vi "Acquire.vi"(8 "error in (no error)":errorcluster, 9 "Data Queue":refnum<queue>, 10 "Data Notifier":refnum<notifier>, 11 "Hardware Resources in":T1) -> (0 "error out":errorcluster, 3 "Hardware Resources out":T1)   [LabVIEW 2016, in "Acquisition.lvlib"]
doc: "Perform the acquisition. Replace the contents of this diagram with calls to acquisition hardware."
uses:
  Acquisition.lvlib
  Hardware Configuration.ctl
  <vilib>/DAQmx/read.llb/DAQmx Read (Analog 1D Wfm NChan NSamp).vi
  <vilib>/DAQmx/miscellaneous.llb/DAQmx Fill In Error Info.vi
  <resource>/objmgr/daqmx.rc
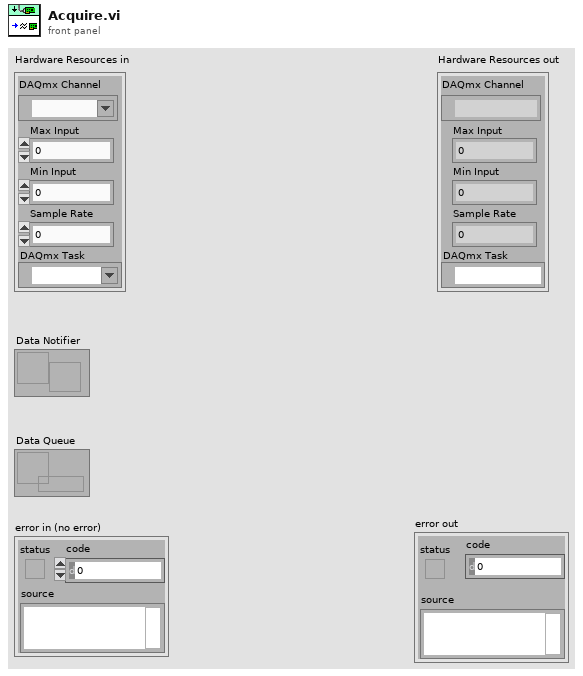
[diagram p1: front panel]
types:
  T1 = typedef "Acquisition.lvlib/Hardware Configuration.ctl" = cluster{"DAQmx Channel":tag, "Max Input":dbl, "Min Input":dbl, "Sample Rate":dbl, "DAQmx Task":refnum<k21>}
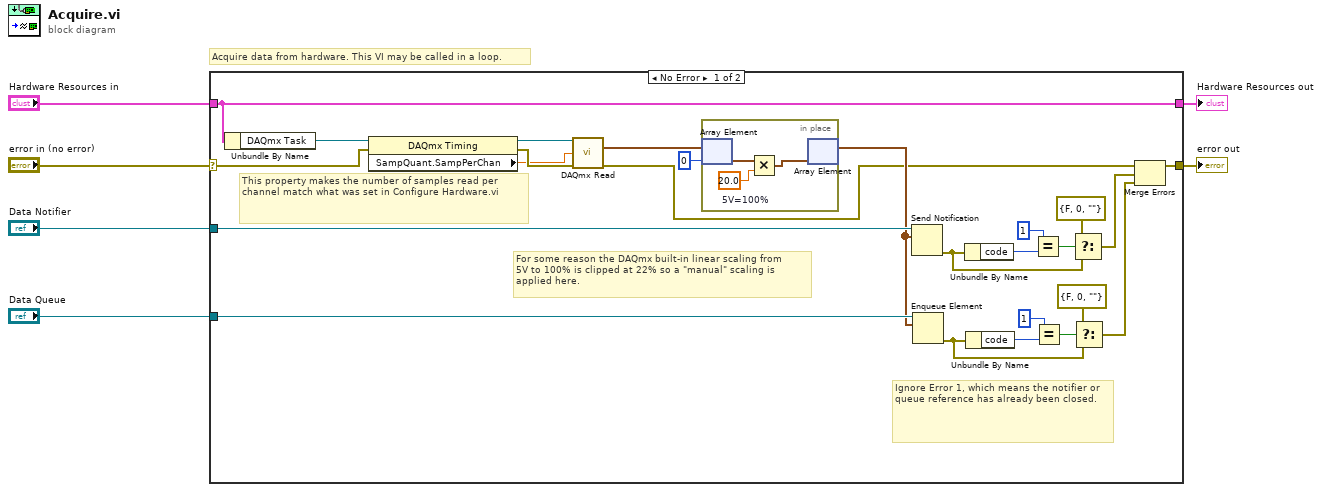
[diagram p0: block diagram]
diagram:
  # "Acquire data from hardware. This VI may be called in a loop."
  n1 = case shown="No Error" "error in (no error)" {
    selector: "error in (no error)" -> [w13 w35]
    tunnel: [w31 w35] -> w5
    tunnel: "Hardware Resources in" -> [w16 w36]
    tunnel: [w16 w36] -> w3
    tunnel: "Data Notifier" -> [w30 _]
    tunnel: "Data Queue" -> [w17 _]
    frame No Error {
      # "For some reason the DAQmx built-in linear scaling from\n5V to 100% is clipped at 22% so a \"manual\" scaling is\napplied here."
      # "This property makes the number of samples read per channel match what was set in Configure Hardware.vi"
      # "Ignore Error 1, which means the notifier or queue reference has already been closed."
      n2 = Unbundle By Name(w16) -> ("DAQmx Task"=w15:refnum<k21>)
      n3 = property class="DAQmx Timing"(reference=w15, error in=w13) -> (reference out=w14:refnum<k21>, error out=w12:errorcluster, "SampQuant.SampPerChan"=w11:dbl)
      n4 = call-poly <vilib>:"DAQmx Read.vi"("task/channels in"=w14, "number of samples per channel"=w11, "error in"=w12) -> ("data"=w9:waveform(dbl)[], "error out"=w7:errorcluster)  [unwired: 10 in, 1 out]
      n5 = in-place {
        w33 = 20.0  # 5V=100%
        n6 = in-place-array #1(w9, 0) -> (w34:waveform(dbl))
        n7 = Multiply(x=w34, y=w33) -> (x*y=w32:waveform(dbl))
        n8 = in-place-array #1(w32) -> (w8:waveform(dbl)[])  [unwired: 1 out]
      }
      n9 = Send Notification(notification=w8, notifier=w30) -> (error out=w26:errorcluster)  [unwired: 1 in, 1 out]
      n10 = Enqueue Element(queue=w17, element=w8) -> (error out=w22:errorcluster)  [unwired: 2 in, 2 out]
      n11 = Unbundle By Name(w26) -> ("code"=w29:i32)
      n12 = Unbundle By Name(w22) -> ("code"=w19:i32)
      n13 = Equal?(x=1, y=w29) -> (x = y?=w27:bool)
      n14 = Equal?(x=1, y=w19) -> (x = y?=w21:bool)
      n15 = Select(t=errorcluster {"status"=FALSE, "code"=0, "source"=""} ("error constant"), s=w27, f=w26) -> (s? t:f=w25:errorcluster)
      n16 = Select(t=errorcluster {"status"=FALSE, "code"=0, "source"=""} ("error constant"), s=w21, f=w22) -> (s? t:f=w18:errorcluster)
      n17 = Merge Errors(w7, w25, w18) -> (w31:errorcluster)
    }
    frame Error {
    }
  }
  "Hardware Resources out" <- w3
  "error out" <- w5
